vi "SPEED.vi"(9 "Baud":u32=2400, 11 "Python in":string) -> (3 "Python out":string="uart.write(b'\\x5A\\x60\\x00\\x09\\x00\\xCC')\n")   [LabVIEW 2016]
panel:
  out "bytes added":u8[](array[numeric])=[90, 96, 0, 9, 0, 204] format="%.0x"
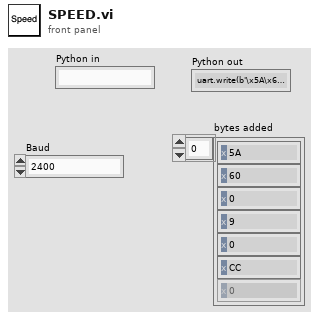
[diagram p1: front panel]
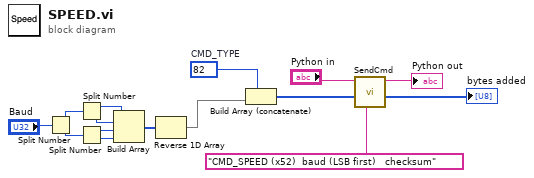
[diagram p0: block diagram]
diagram:
  w15 = u8 82  # CMD_TYPE
  n1 = Split Number(x="Baud") -> (hi(x)=w8:u16, lo(x)=w9:u16)
  n2 = Split Number(x=w8) -> (hi(x)=w7:u8, lo(x)=w6:u8)
  n3 = Split Number(x=w9) -> (hi(x)=w5:u8, lo(x)=w4:u8)
  n4 = Build Array(w7, w6, w5, w4) -> (w3:u8[])
  n5 = Reverse 1D Array(array=w3) -> (reversed array=w2:u8[])
  n6 = Build Array (concatenate)(w15, w2) -> (w12:u8[])
  n7 = call "SendCmd.vi"("Comment"="CMD_SPEED (x52)  baud (LSB first)   checksum", "Array In"=w12, "Python in"="Python in") -> ("Array Sent"=→"bytes added":u8[], "Python out"=→"Python out":string)  [unwired: 7 in]
